vi "NS Write.vi"(8 "error in":errorcluster, 10 "Data":variant, 11 "Message":string) -> (0 "error out":errorcluster)   [LabVIEW 2020]
uses:
  Globals/Phase III Globals.vi
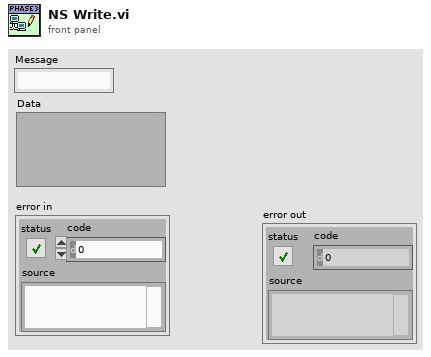
[diagram p1: front panel]
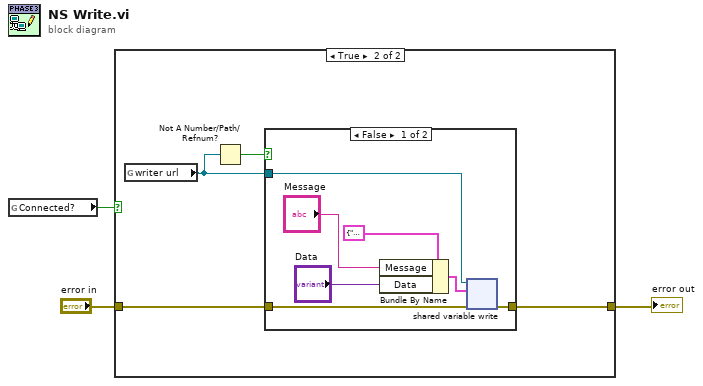
[diagram p0: block diagram]
diagram:
  n1 = global read "Phase III Globals.vi" "Connected?"() -> (w3:bool)
  n2 = case shown="True" w3 {
    tunnel: "error in" -> [w4 w7]
    tunnel: [w4 w6] -> w1
    frame False {
    }
    frame True {
      n3 = global read "Phase III Globals.vi" "writer url"() -> (w5:refnum<k21>)
      n4 = Not A Number/Path/Refnum?(number/path/refnum=w5) -> (NaN/Path/Refnum?=w8:bool)
      n5 = case shown="False" w8 {
        tunnel: w5 -> [w15 _]
        tunnel: w7 -> [w10 w16]
        tunnel: [w9 w16] -> w6
        frame False {
          n6 = Bundle By Name(cluster=cluster{"Message":string, "Data":variant} {"Message"="", "Data"=variant}, "Message"="Message", "Data"="Data") -> (w14:cluster{"Message":string, "Data":variant})
          n7 = shared-variable-write(w15, w10, w14) -> (w9:errorcluster)  [unwired: 1 in, 2 out]
        }
        frame True {
        }
      }
    }
  }
  "error out" <- w1
